vi "Read Data_HoldingRegistors.vi"(8 "error in (no error)":errorcluster, 11 "Device in":refnum<class "RS232_Device.lvclass">) -> (0 "error out":errorcluster, 2 "register values":dbl[](array[numeric]), 3 "Device out":refnum<class "RS232_Device.lvclass">)   [LabVIEW 2023, in "RS232_Device.lvclass"]
uses:
  RS232_Device.lvclass
  D:/SamparkProdLine/subVIs/DAQ Device/Modbus_Device/DAQ_Device.lvclass
  RS232_Device.lvclass/RS232_Device.ctl
panel:
  out "resulting string":string
  out "Response":string
  out "return count":u32
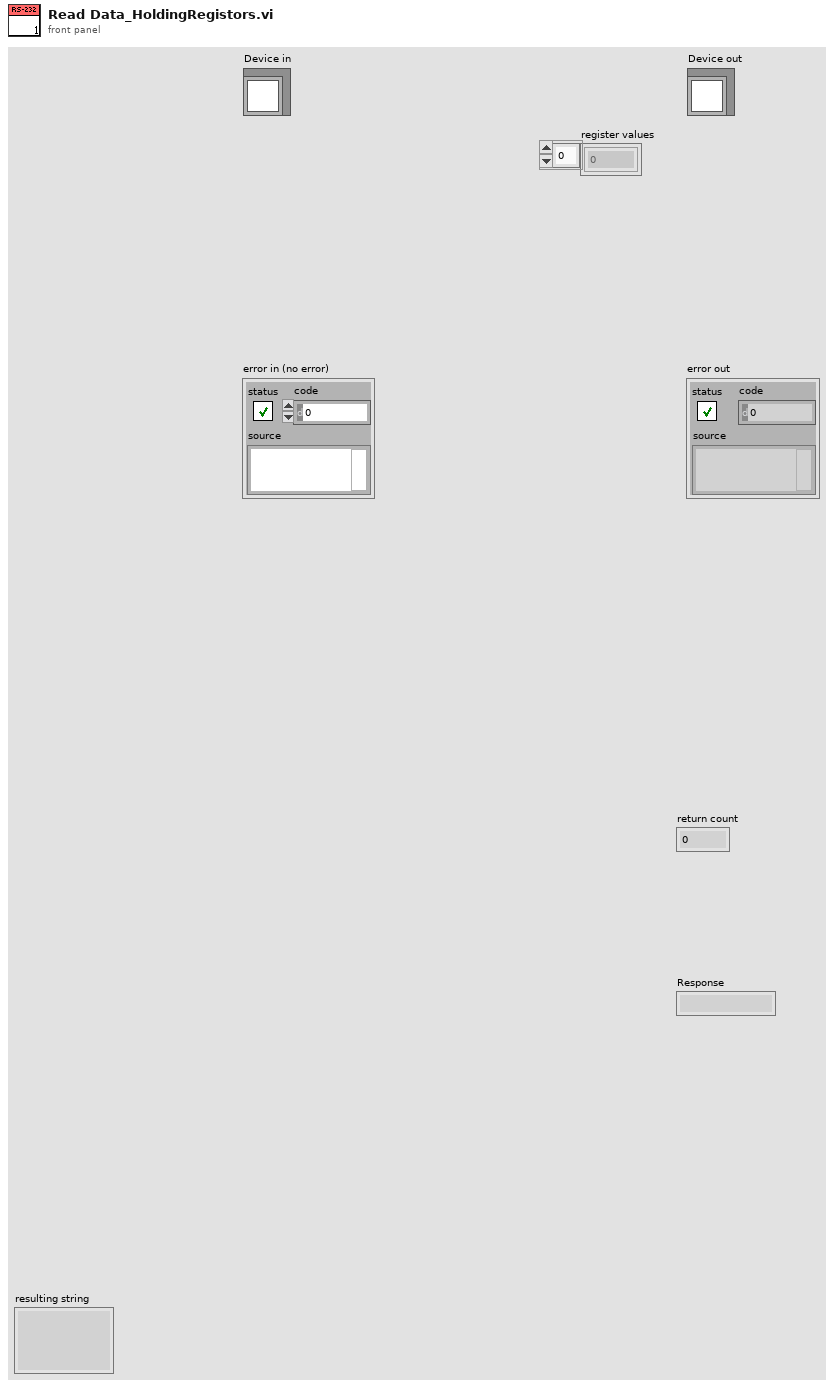
[diagram p1: front panel]
types:
  T1 = typedef "DAQ Device_IO ChannelsData.ctl" = cluster{"#DigitalInputs":u16, "StartAddress_DI":u16, "#DigitalOutputs":u16, "StartAddress_DO":u16, "#AnalogInputs":u16, "StartAddress_AI":u16, "#AnalogOutputs":u16, "StartAddress_AO":u16, "Coil_ReadData":bool[], "Coil_WriteData":bool[], "AI_Data":u16[], "AO_Data":u16[]}
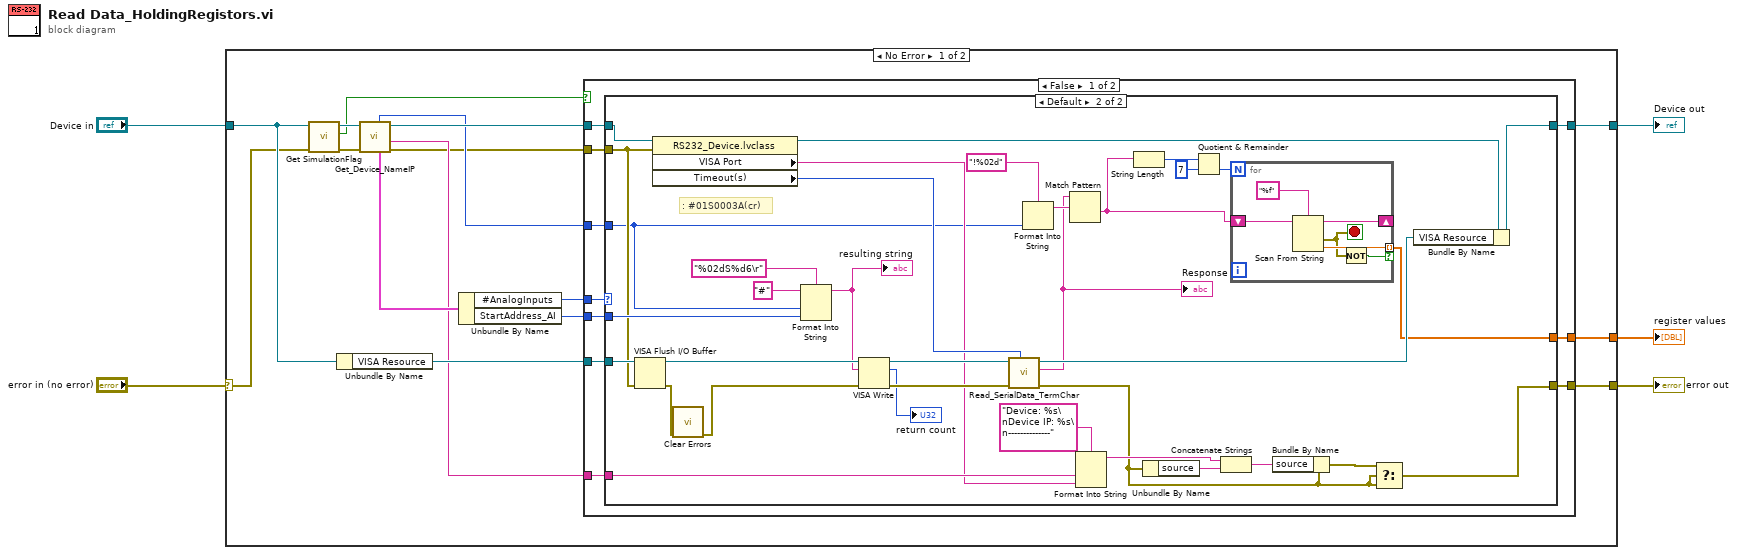
[diagram p0: block diagram]
diagram:
  n1 = case shown="No Error" "error in (no error)" {
    selector: "error in (no error)" -> [w9 w78]
    tunnel: [w20 w78] -> w1
    tunnel: [w21 w77] -> w3
    tunnel: "Device in" -> [w13 w77]
    tunnel: [w18 _] -> w2
    frame No Error {
      n2 = call-dynamic "Get SimulationFlag.vi"("error in (no error)"=w9, "Device in"=w13) -> ("error out"=w17:errorcluster, "Simulation?"=w10:bool, "Device out"=w14:refnum<class "RS232_Device.lvclass">)  [unwired: 7 in]
      n3 = Unbundle By Name(w13) -> ("VISA Resource"=w19:refnum<visa-resource-name>)
      n4 = call-dynamic "Get_Device_NameIP.vi"("error in (no error)"=w17, "Device in"=w14) -> ("error out"=w8:errorcluster, "Device Name"=w11:string, "Device out"=w15:refnum<class "RS232_Device.lvclass">, "IO Channels"=w16:T1, "Unit ID"=w12:u8)  [unwired: 4 in, 1 out]
      n5 = Unbundle By Name(w16) -> ("#AnalogInputs"=w6:u16, "StartAddress_AI"=w7:u16)
      n6 = case shown="False" w10 {
        tunnel: [w31 w76] -> w21
        tunnel: [w30 w75] -> w20
        tunnel: w19 -> [w29 _]
        tunnel: w15 -> [w26 w76]
        tunnel: w11 -> [w28 _]
        tunnel: [w23 _] -> w18
        tunnel: w12 -> [w24 _]
        tunnel: w7 -> [w27 _]
        tunnel: w8 -> [w25 w75]
        tunnel: w6 -> [w22 _]
        frame False {
          n7 = case shown="Default" w22 {
            tunnel: [w33 w68] -> w31
            tunnel: [w32 w67] -> w30
            tunnel: w29 -> [_ w66]
            tunnel: w28 -> [_ w65]
            tunnel: w27 -> [_ w50]
            tunnel: w26 -> [w33 w46]
            tunnel: w25 -> [w32 w45]
            tunnel: w24 -> [_ w42]
            tunnel: [_ w34] -> w23
            frame 0 {
            }
            frame Default {
              # ": #01S0003A(cr)"
              n8 = VISA Flush I/O Buffer(VISA resource name=w66, error in (no error)=w45) -> (VISA resource name out=w59:refnum<visa-resource-name>, error out=w58:errorcluster)  [unwired: 1 in]
              n9 = property class="RS232_Device.lvclass"(reference=w46, error in=w45) -> (reference out=w47:refnum<class "RS232_Device.lvclass">, "VISA Port"=w43:string, "Timeout(s)"=w44:i32)  [unwired: 1 out]
              n10 = call <vilib>:"Clear Errors.vi"("error in (no error)"=w58) -> ("error out"=w57:errorcluster)  [unwired: 5 in, 1 out]
              n11 = Format Into String(format string="%02dS%d6\r", initial string="#", w42, w50) -> (resulting string=w49:string)  [unwired: 1 in, 1 out]
              "resulting string" <- w49
              n12 = VISA Write(VISA resource name=w59, write buffer=w49, error in (no error)=w57) -> (VISA resource name out=w56:refnum<visa-resource-name>, return count=→"return count":u32, error out=w55:errorcluster)
              n13 = call "Read_SerialData_TermChar.vi"("timeout (50ms)"=w44, "error in (no error)"=w55, "VISA Refnum in"=w56) -> ("error out"=w54:errorcluster, "StringData"=w40:string, "VISA Refnum out"=w53:refnum<visa-resource-name>)  [unwired: 6 in]
              "Response" <- w40
              n14 = Format Into String(format string="!%02d" ("regular expression"), w42) -> (resulting string=w41:string)  [unwired: 2 in, 1 out]
              n15 = Match Pattern(string=w40, regular expression=w41) -> (after substring=w36:string)  [unwired: 1 in, 3 out]
              n16 = Format Into String(format string="Device: %s\nDevice IP: %s\n--------------", w65, w43) -> (resulting string=w61:string)  [unwired: 2 in, 1 out]
              n17 = String Length(string=w36) -> (length=w38:i32)
              n18 = Unbundle By Name(w54) -> ("source"=w63:string)
              n19 = Quotient & Remainder(x=w38, y=7) -> (floor(x/y)=w35:i32)  [unwired: 1 out]
              n20 = Concatenate Strings(w61, w63) -> (w60:string)
              n21 = for {
                N: w35 -> [_]
                shift-right: [w72] -> _
                shift-left: w36 -> [w74]
                tunnel: [w71] -> w34 mode=indexing if=w69
                stop <- w70 stop-if-true
                n22 = Scan From String(format string="%f", input string=w74) -> (remaining string=w72:string, error out=w70:errorcluster, output 1=w71:dbl)  [unwired: 3 in, 1 out]
                n23 = Not(x=w70) -> (.not. x?=w69:bool)
              }
              n24 = Bundle By Name(cluster=w54, "source"=w60) -> (w64:errorcluster)
              n25 = Select(t=w64, s=w54, f=w54) -> (s? t:f=w67:errorcluster)
              n26 = Bundle By Name(cluster=w47, "VISA Resource"=w53) -> (w68:refnum<class "RS232_Device.lvclass">)
            }
          }
        }
        frame True {
        }
      }
    }
    frame Error {
    }
  }
  "error out" <- w1
  "Device out" <- w3
  "register values" <- w2
